vi "Example 3D Plot (Torus).vi"() -> ()   [LabVIEW 2010]
uses:
  <vilib>/Math Plots/3D Math Plots/3D Surface/3D Surface XCtrl/3D Surface.xctl
  <vilib>/Math Plots/3D Math Plots/3D Surface/3D Surface Datatype/Public/Plot Helper (Matrix).vi
  <vilib>/Math Plots/3D Math Plots/3D Surface/3D Surface Datatype/3D Surface Datatype.lvclass
panel:
  in  "Inner Radius C":dbl(slide) scale=0.0..5.0
  in  "Tube Radius A":dbl(slide) scale=1e-06..5.0
  out "3D Surface":refnum<class "3D Plot Datatype.lvclass">[](xcontrol)
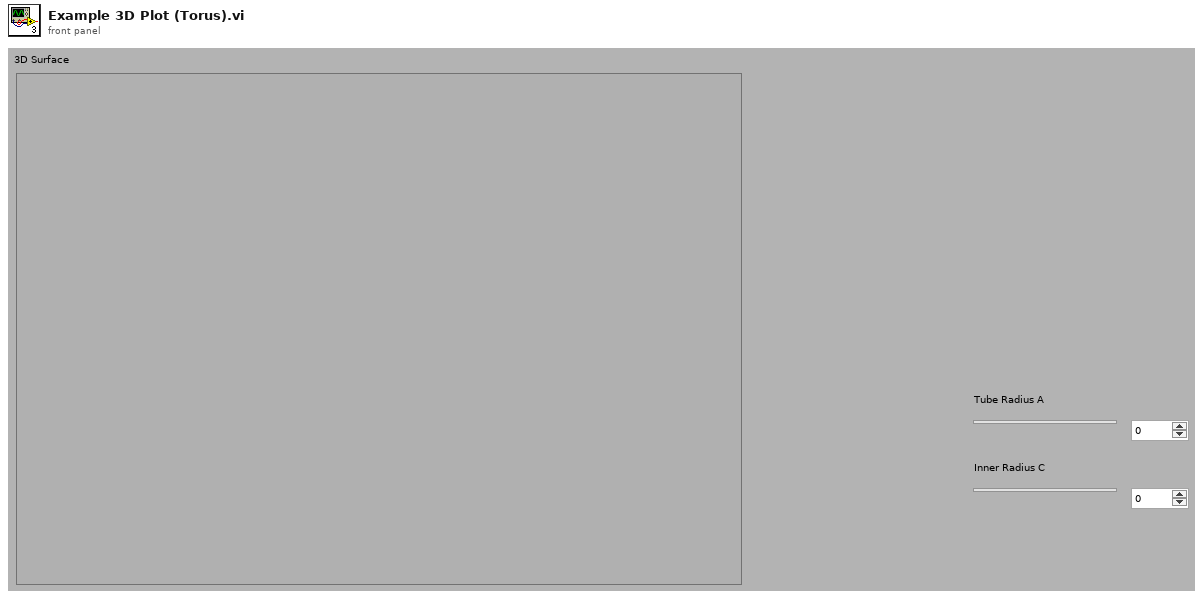
[diagram p1: front panel]
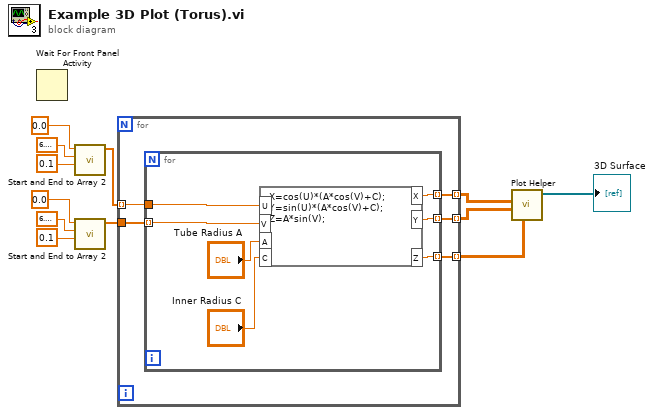
[diagram p0: block diagram]
diagram:
  n1 = Wait For Front Panel Activity() -> ()  [unwired: 3 in, 1 out]
  n2 = call "Start and End to Array 2.vi"("Step or # Pts"=0.1, "End"=6.283185307179586, "Start"=0.0) -> ("Array"=w11:dbl[])  [unwired: 8 in]
  n3 = call "Start and End to Array 2.vi"("Step or # Pts"=0.1, "End"=6.283185307179586, "Start"=0.0) -> ("Array"=w10:dbl[])  [unwired: 8 in]
  n4 = for {
    tunnel: w11 -> [w16] mode=indexing
    tunnel: w10 -> [w17]
    tunnel: [w15] -> w3 mode=indexing
    tunnel: [w14] -> w2 mode=indexing
    tunnel: [w13] -> w1 mode=indexing
    n5 = for {
      tunnel: w17 -> [w21] mode=indexing
      tunnel: w16 -> [w22]
      tunnel: [w20] -> w15 mode=indexing
      tunnel: [w19] -> w14 mode=indexing
      tunnel: [w18] -> w13 mode=indexing
      n6 = formula code="X=cos(U)*(A*cos(V)+C);\nY=sin(U)*(A*cos(V)+C);\nZ=A*sin(V);"("U"=w22, "V"=w21, "A"="Tube Radius A", "C"="Inner Radius C") -> ("Z"=w18:dbl, "X"=w20:dbl, "Y"=w19:dbl)
    }
  }
  n7 = call-poly <vilib>:"Plot Helper.vi"("z matrix"=w1, "y matrix"=w2, "x matrix"=w3) -> ("3D Plot lvclass Array out"=→"3D Surface":refnum<class "3D Plot Datatype.lvclass">[])  [unwired: 3 in, 5 out]
